vi "reset_main_panel.vi"(6 "Iteration":refnum<vi>, 8 "Working Directory":refnum<vi>, 9 "Active Element":refnum<vi>, 10 "Simulation Log":refnum<vi>, 11 "Plant Structure":refnum<vi>) -> ()   [LabVIEW 2019]
uses:
  lib/libSimulationControl/libSimulationControl.lvlib
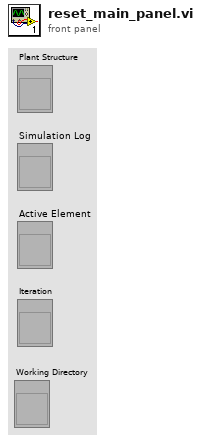
[diagram p1: front panel]
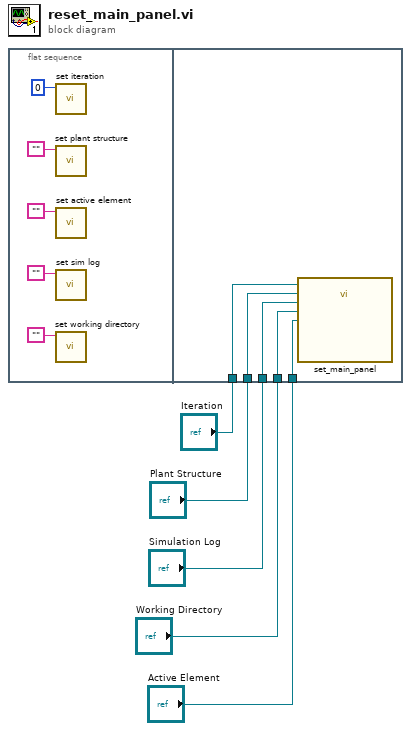
[diagram p0: block diagram]
diagram:
  n1 = flat-sequence {
    tunnel: "Plant Structure" -> [w15]
    tunnel: "Simulation Log" -> [w14]
    tunnel: "Active Element" -> [w13]
    tunnel: "Iteration" -> [w12]
    tunnel: "Working Directory" -> [w11]
    frame #0 {
      n2 = call "set iteration.vi"("iter"=0 ("Value")) -> ()  [unwired: 10 in, 1 out]
      n3 = call "set plant structure.vi"("structure"="") -> ()  [unwired: 10 in, 1 out]
      n4 = call "set active element.vi"("elem"="") -> ()  [unwired: 10 in, 1 out]
      n5 = call "set sim log.vi"("log"="") -> ()  [unwired: 10 in, 1 out]
      n6 = call "set working directory.vi"("dir"="") -> ()  [unwired: 10 in, 1 out]
    }
    frame #1 {
      n7 = call "set_main_panel.vi"("Active Element"=w13, "Working Directory"=w11, "Simulation Log"=w14, "Plant Structure"=w15, "Iteration"=w12) -> ()  [unwired: 7 in]
    }
  }
